vi "Append VI List of Controls to Report (string).vi"(0 "report in":refnum<class "NI_report.lvclass">, 1 "include only controls in con pane?":bool, 2 "image format (jpeg)":enum32{"PNG", "JPEG", "GIF"}(ring)=enum."JPEG", 5 "VI":string, 7 "alignment (default)":T2, 11 "error in (no error)":errorcluster, 12 "include control descriptions?":bool, 13 "include control data types?":bool, 14 "MS Office parameters":T1) -> (4 "report out":refnum<class "NI_report.lvclass">, 6 "VI name out":string, 8 "start out (Word)":i32, 10 "end out (Word)":i32, 15 "error out":errorcluster)   [LabVIEW 2017, in "NI_ReportGenerationCore.lvlib"]
doc: "Appends a list of controls and indicators of the VI you specify in <B>VI</B> to a report. Wire data to the <B>VI</B> input to determine the polymorphic instance to use or manually select the instance."
uses:
  <vilib>/Utility/NIReport.llb/NI_ReportGenerationCore.lvlib
  <vilib>/Utility/NIReport.llb/NI_report.lvclass
  <vilib>/Utility/NIReport.llb/HTML Report Image Alignment.ctl
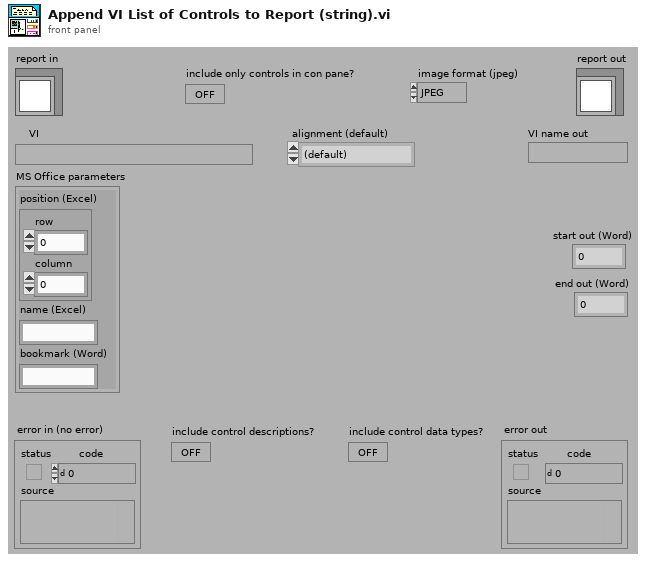
[diagram p1: front panel]
types:
  T1 = cluster{"position (Excel)":cluster{"row":i32, "column":i32}, "name (Excel)":string, "bookmark (Word)":string}
  T2 = typedef "NI_ReportGenerationCore.lvlib/HTML Report Image Alignment.ctl" = enum16{"(default)", "LEFT", "RIGHT", "TOP", "TEXTTOP", "MIDDLE", "ABSMIDDLE", "BASELINE", "BOTTOM", "ABSBOTTOM"}
  T3 = enum32{"invalid app kind", "Development System", "Run Time System", "Student Edition", "Embedded LabVIEW", "Evaluation", "Custom"}
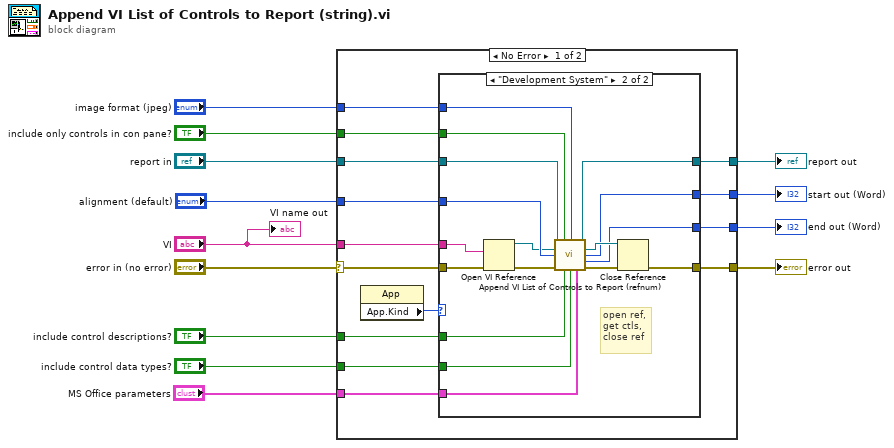
[diagram p0: block diagram]
diagram:
  n1 = case shown="No Error" "error in (no error)" {
    selector: "error in (no error)" -> [w23 w48]
    tunnel: [w19 w48] -> w7
    tunnel: "include control descriptions?" -> [w27 _]
    tunnel: "include control data types?" -> [w26 _]
    tunnel: "report in" -> [w18 w47]
    tunnel: "image format (jpeg)" -> [w25 _]
    tunnel: "include only controls in con pane?" -> [w24 _]
    tunnel: "VI" -> [w22 _]
    tunnel: "alignment (default)" -> [w21 _]
    tunnel: "MS Office parameters" -> [w20 _]
    tunnel: [w17 _] -> w3
    tunnel: [w16 w47] -> w2
    tunnel: [w15 _] -> w1
    frame No Error {
      n2 = property class="App"() -> ("App.Kind"=w14:T3)  [unwired: 2 in, 2 out]
      n3 = case shown="\"Development System\"" w14 {
        tunnel: w27 -> [_ w46]
        tunnel: w26 -> [_ w45]
        tunnel: w25 -> [_ w44]
        tunnel: w24 -> [_ w43]
        tunnel: w23 -> [w28 w42]
        tunnel: w22 -> [_ w40]
        tunnel: w21 -> [_ w39]
        tunnel: w20 -> [_ w38]
        tunnel: [w28 w35] -> w19
        tunnel: w18 -> [w29 w33]
        tunnel: [_ w32] -> w17
        tunnel: [w29 w31] -> w16
        tunnel: [_ w30] -> w15
        frame "invalid app kind", Default {
        }
        frame "Development System" {
          # "open ref,\nget ctls,\nclose ref"
          n4 = Open VI Reference(vi path=w40, error in (no error)=w42) -> (vi reference=w34:refnum<vi>, error out=w41:errorcluster)  [unwired: 4 in]
          n5 = call <vilib>:"Append VI List of Controls to Report (refnum).vi"("report in"=w33, "include only controls in con pane?"=w43, "image format (jpeg)"=w44, "VI"=w34, "alignment (default)"=w39, "error in (no error)"=w41, "include control descriptions?"=w46, "include control data types?"=w45, "MS Office parameters"=w38) -> ("report out"=w31:refnum<class "NI_report.lvclass">, "VI out"=w36:refnum<vi>, "start out (Word)"=w32:i32, "end out (Word)"=w30:i32, "error out"=w37:errorcluster)  [unwired: 2 in]
          n6 = Close Reference(reference=w36, error in (no error)=w37) -> (error out=w35:errorcluster)
        }
      }
    }
    frame Error {
    }
  }
  "error out" <- w7
  "report out" <- w2
  "start out (Word)" <- w3
  "end out (Word)" <- w1
  "VI name out" <- "VI"
